vi "PRL Read Queue.vi"(11 "timeout in ms (5)":i32=5) -> (0 "Has Data?":bool, 1 "Digital Values":bool[][](array[boolean]), 2 "Analog Values":sgl[][](array[numeric]), 3 "Phasor Values":csg[][](array[numeric]), 5 "Timestamp Values":timestamp[](array[timestamp]))   [LabVIEW 2018, in "S3DK.lvlib" / "PMU Recorder Light.lvlib"]
uses:
  PMU Recorder Light.lvlib
panel:
  out "error out":errorcluster
  in  "error in (no error)":errorcluster
  # "INPUT"
  # "INTERMEDIATE"
  # "OUTPUT"
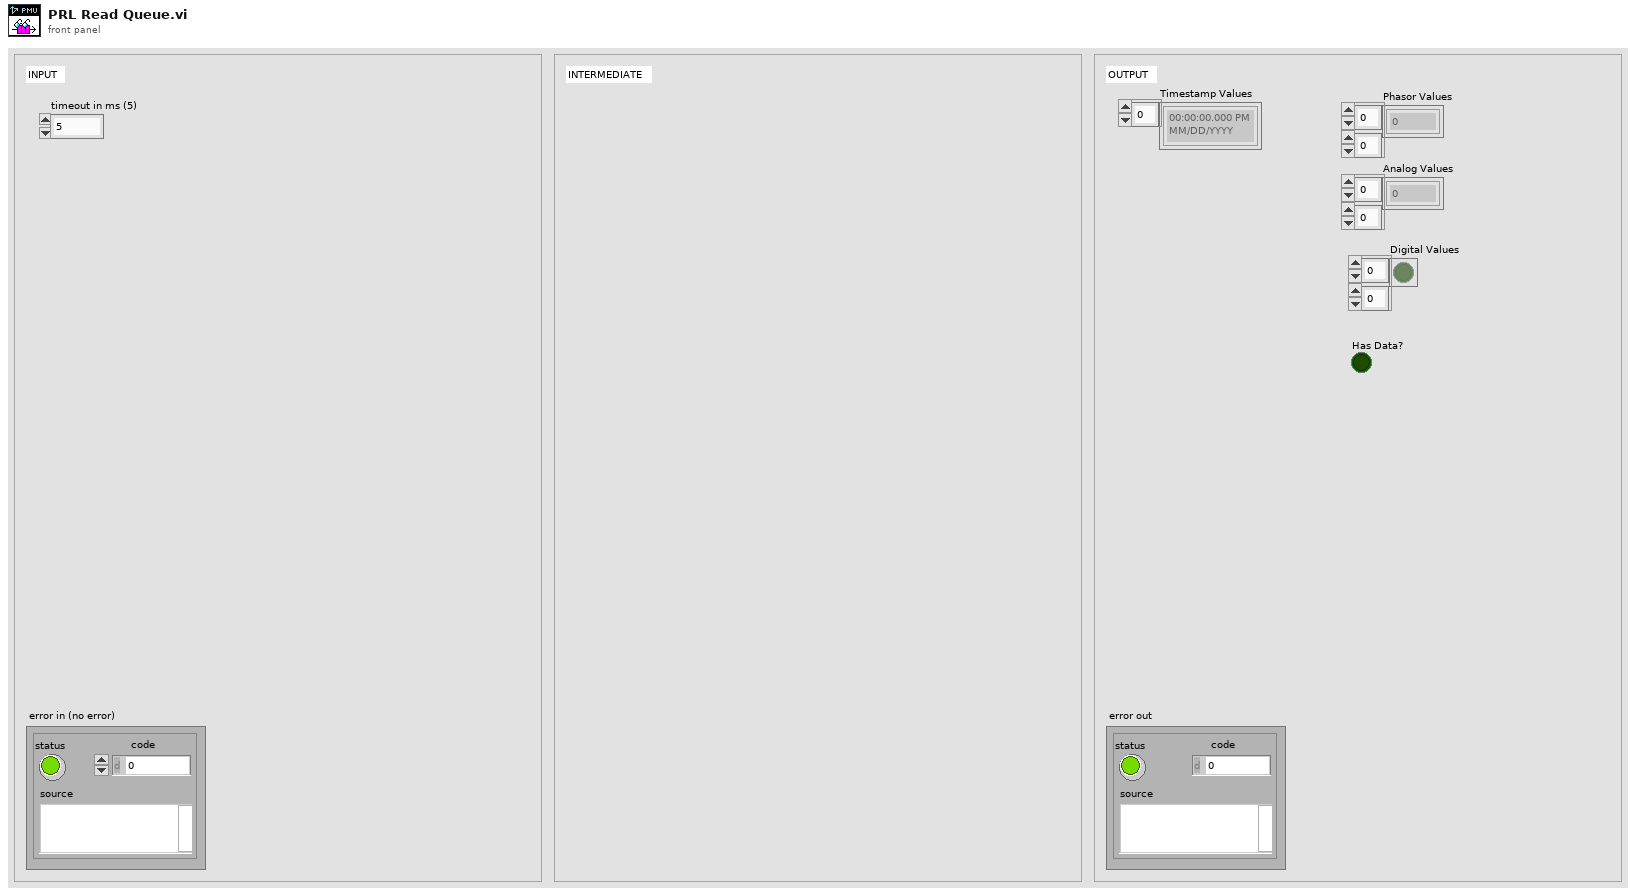
[diagram p1: front panel]
types:
  T1 = cluster{"Timestamp Values":timestamp[], "Phasor Values":csg[][], "Analog Values":sgl[][], "Digital Values":bool[][], "System Data Buffer":sgl[][]}
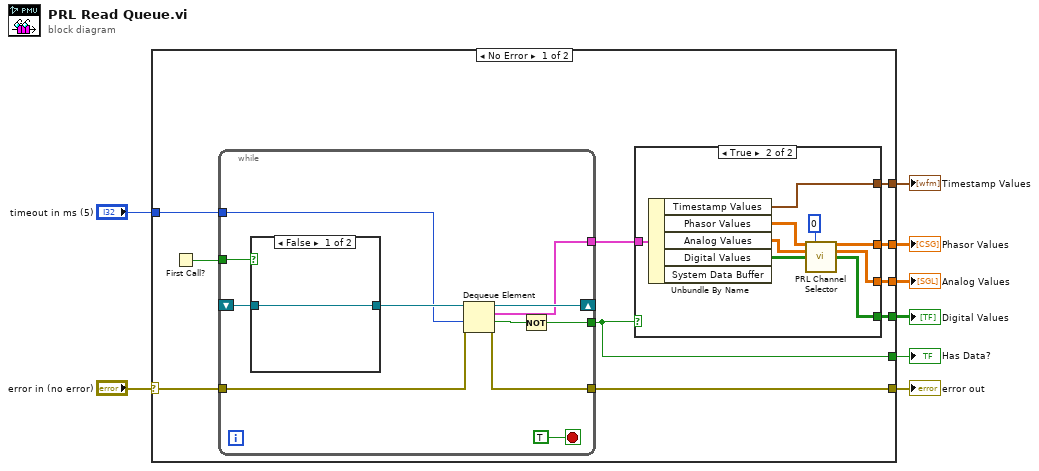
[diagram p0: block diagram]
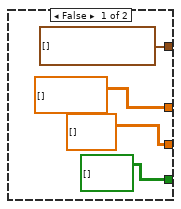
[diagram p2: hidden frame]
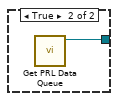
[diagram p3: hidden frame]
diagram:
  n1 = case shown="No Error" "error in (no error)" {
    selector: "error in (no error)" -> [w10 w45]
    tunnel: "timeout in ms (5)" -> [w17 _]
    tunnel: [w15 _] -> w7
    tunnel: [w14 _] -> w6
    tunnel: [w13 _] -> w5
    tunnel: [w12 _] -> w4
    tunnel: [w9 w45] -> w2
    tunnel: [w11 _] -> w1
    frame No Error {
      n2 = First Call?() -> (First Call?: T/F=w18:bool)
      n3 = while {
        tunnel: w18 -> [w41]
        shift-right: [w38] -> _
        shift-left: _ -> [w40]
        tunnel: w17 -> [w37]
        tunnel: [w35] -> w11
        tunnel: [w34] -> w16
        tunnel: w10 -> [w33]
        tunnel: [w32] -> w9
        stop <- TRUE stop-if-true
        n4 = case shown="False" w41 {
          tunnel: w40 -> [w43 _]
          tunnel: [w43 w44] -> w39
          frame False {
          }
          frame True {
            n5 = call "Get PRL Data Queue.vi"() -> ("PRL Data Queue"=w44:refnum<queue>)  [unwired: 11 in]
          }
        }
        n6 = Dequeue Element(queue=w39, timeout in ms (-1)=w37, error in (no error)=w33) -> (queue out=w38:refnum<queue>, element=w34:T1, timed out?=w36:bool, error out=w32:errorcluster)
        n7 = Not(x=w36) -> (.not. x?=w35:bool)
      }
      n8 = case shown="True" w11 {
        tunnel: w16 -> [_ w31]
        tunnel: [csg[][] [] ("Phasor Values Out") w27] -> w15
        tunnel: [sgl[][] [] ("Analog Values Out") w26] -> w14
        tunnel: [bool[][] [] ("Digital Values Out") w25] -> w13
        tunnel: [timestamp[] [] ("Timestamp Values") w23] -> w12
        frame False {
        }
        frame True {
          n9 = Unbundle By Name(w31) -> ("Timestamp Values"=w23:timestamp[], "Phasor Values"=w30:csg[][], "Analog Values"=w29:sgl[][], "Digital Values"=w28:bool[][])  [unwired: 1 out]
          n10 = call "PRL Channel Selector.vi"("Phasor Values In"=w30, "Cut Index"=0, "Analog Values In"=w29, "Digital Values In"=w28) -> ("Phasor Values Out"=w27:csg[][], "Analog Values Out"=w26:sgl[][], "Digital Values Out"=w25:bool[][])  [unwired: 8 in, 1 out]
        }
      }
    }
    frame Error {
    }
  }
  "Phasor Values" <- w7
  "Analog Values" <- w6
  "Digital Values" <- w5
  "Timestamp Values" <- w4
  "error out" <- w2
  "Has Data?" <- w1
